vi "Color detection.vi"() -> ()   [LabVIEW 2015]
uses:
  <vilib>/MakerHub/LINX/Public/Peripherals/Digital/Digital Write 1 Chan.vi
  <vilib>/MakerHub/LINX/Public/Peripherals/Digital/Digital Write N Chans.vi
  <vilib>/MakerHub/LINX/Private/Local IO/LinxDigitalWrite.vi
  <vilib>/MakerHub/LINX/Public/Utilities/Check Channel.vi
  <vilib>/MakerHub/LINX/Public/Utilities/Open Serial.vi
  <vilib>/MakerHub/LINX/Private/Utilties/Generate Error.vi
  <vilib>/vision/NI_Vision_Development_Module.lvlib
  <vilib>/MakerHub/LINX/LMH-LINX.lvlib
panel:
  in  "Green OutPin":u8
  in  "Blue Outpin":u8
  in  "Red OutPin":u8
  in  "Serial Port":refnum<visa-resource-name>="N/A"
  out "Green":bool
  out "Blue":bool
  out "Red":bool
  out "Image":T1(plugin-control)
  in  "Rectangle":T2 {"Rotation" min=-90.0 max=90.0 step=1.0 format="%.2f"; "Left" scale=0.0..1024.0; "Right" scale=0.0..1024.0}
  in  "stop":bool
  out "Color Spectrum":dbl[](array[numeric]) format="%.2f"
  in  "Image Type":T3 items=["Grayscale (U8)", "Grayscale (I16)", "Grayscale (SGL)", "Complex (CSG)", "RGB (U32)", "HSL (U32)", "RGB (U64)", "Grayscale (U16)"]
  in  "File Path":path
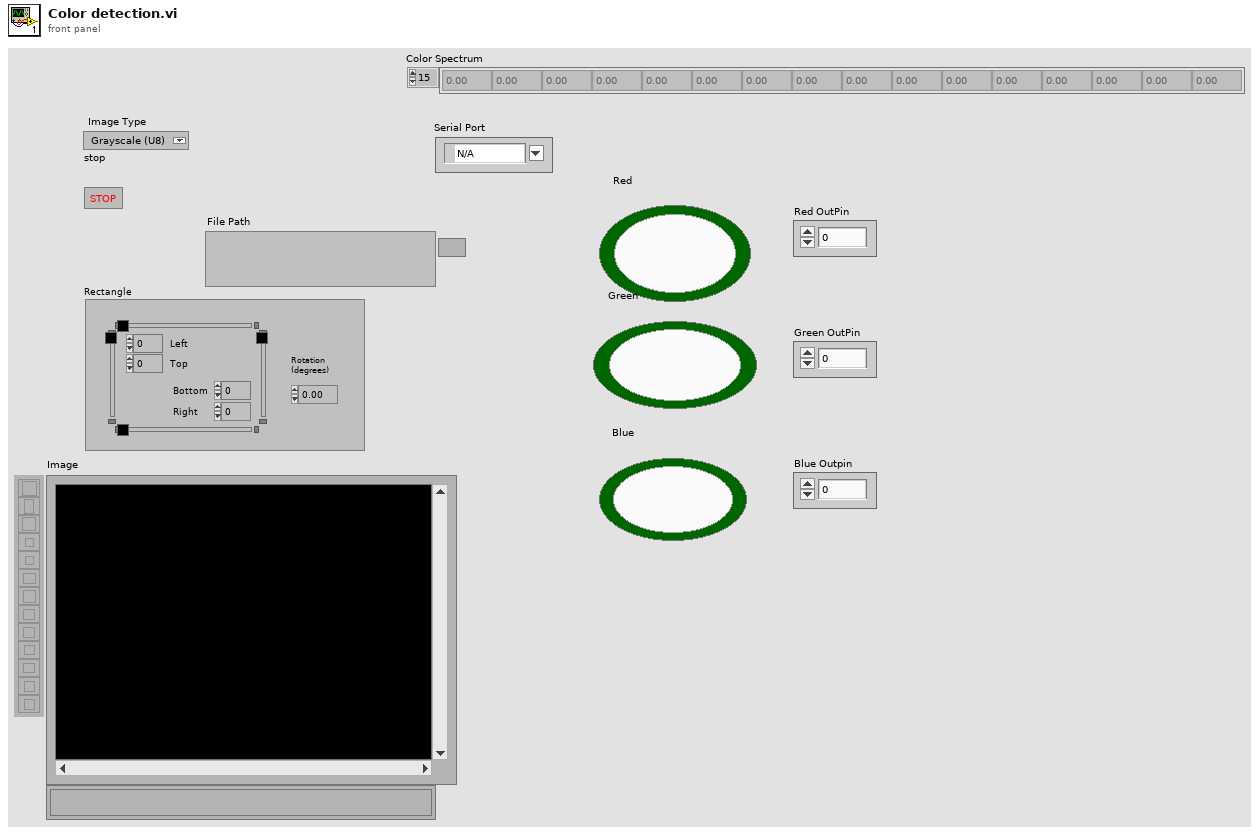
[diagram p1: front panel]
types:
  T1 = typedef "IMAQ Image.ctl" = refnum<image>
  T2 = typedef "IMAQ Rectangle" = cluster{"Left":i32, "Top":i32, "Right":i32, "Bottom":i32, "Rotation":dbl}
  T3 = typedef "Image Type" = u32
  T4 = typedef "LMH-LINX.lvlib/LINX Ref.ctl" = cluster{"IO":T5, "Interface":T6, "LINX Device Config":T7}
  T5 = typedef "LMH-LINX.lvlib/Platform.ctl" = enum16{"Remote", "Local"}
  T6 = typedef "LMH-LINX.lvlib/Interface.ctl" = enum16{"Serial", "TCP"}
  T7 = typedef "LMH-LINX.lvlib/Device.lvlib/LINX Device Config.ctl" = cluster{"Interface":T6, "COM Port":refnum<visa-resource-name>, "TCP Configuration":T8, "Device Family":u8, "Device ID":u8, "Device Name":string, "TCP Ref":refnum<k5>, "Channels":T9}
  T8 = typedef "LMH-LINX.lvlib/Device.lvlib/TCP Config.ctl" = cluster{"IP Address":string, "Port":u16}
  T9 = typedef "LMH-LINX.lvlib/Channels.ctl" = cluster{"DI":u8[], "DO":u8[], "AI":u8[], "AO":u8[], "PWM":u8[], "QE":u8[], "UART":u8[], "I2C 2":u8[], "SPI":u8[], "CAN":u8[], "Servo":u8[], "AI Ref (V)":dbl, "AI Resolution (Bits)":u8, "AO Ref (V)":dbl, "AO Resolution (Bits)":u8}
  T10 = typedef "ROI Descriptor" = cluster{"Global Rectangle":i32[], "Contours":cluster{"ID":enum32{"External", "Internal"}, "Type":u32, "Coordinates":i32[]}[]}
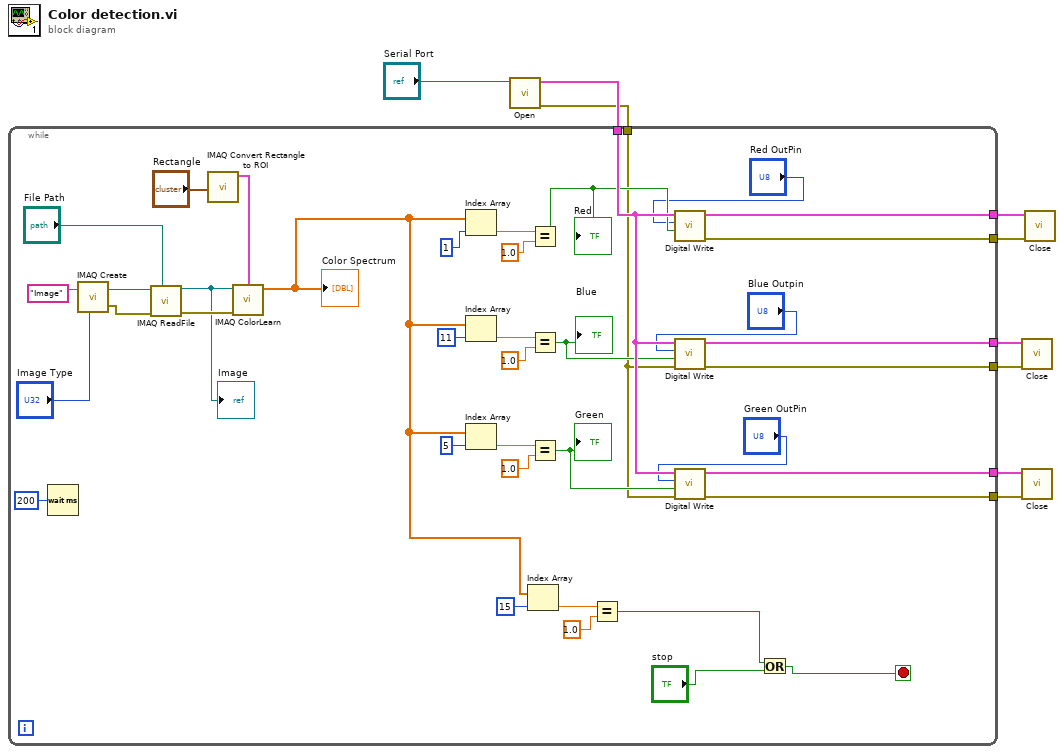
[diagram p0: block diagram]
diagram:
  n1 = call-poly <vilib>:"Open.vi"("Serial Port"="Serial Port") -> ("Error Out"=w7:errorcluster, "LINX Resource"=w8:T4)  [unwired: 8 in, 1 out]
  n2 = while {
    tunnel: w8 -> [w30]
    tunnel: w7 -> [w23]
    tunnel: [w22] -> w6
    tunnel: [w21] -> w5
    tunnel: [w20] -> w4
    tunnel: [w19] -> w3
    tunnel: [w18] -> w2
    tunnel: [w17] -> w1
    stop <- w10 stop-if-true
    n3 = Wait (ms)(milliseconds to wait=u32 200) -> ()  [unwired: 1 out]
    n4 = call "IMAQ Create"("Image Name"="Image", "Image Type"="Image Type") -> ("New Image"=w48:T1, "error out"=w47:errorcluster)  [unwired: 3 in]
    n5 = call "IMAQ ReadFile"("File Path"="File Path", "error in (no error)"=w47, "Image"=w48) -> ("error out"=w43:errorcluster, "Image Out"=w40:T1)  [unwired: 4 in, 3 out]
    "Image" <- w40
    n6 = call "IMAQ Convert Rectangle to ROI"("Rectangle"="Rectangle") -> ("ROI Descriptor"=w42:T10)  [unwired: 8 in, 1 out]
    n7 = call "IMAQ ColorLearn"("ROI Descriptor"=w42, "Image"=w40, "error in (no error)"=w43) -> ("Color Spectrum"=w13:dbl[])  [unwired: 5 in, 1 out]
    "Color Spectrum" <- w13
    n8 = Index Array(array=w13, index=1) -> (element=w38:dbl)
    n9 = Index Array(array=w13, index=11) -> (element=w35:dbl)
    n10 = Index Array(array=w13, index=5) -> (element=w32:dbl)
    n11 = Index Array(array=w13, index=15) -> (element=w15:dbl)
    n12 = Equal?(x=w38, y=1.0) -> (x = y?=w29:bool)
    "Red" <- w29
    n13 = Equal?(x=w35, y=1.0) -> (x = y?=w25:bool)
    "Blue" <- w25
    n14 = Equal?(x=w32, y=1.0) -> (x = y?=w28:bool)
    "Green" <- w28
    n15 = Equal?(x=w15, y=1.0) -> (x = y?=w12:bool)
    n16 = call-poly <vilib>:"Digital Write.vi"("Output Value"=w29, "DO Channel"="Red OutPin", "LINX Resource"=w30) -> ("Error Out"=w21:errorcluster, "LINX Resource"=w22:T4)  [unwired: 7 in]
    n17 = call-poly <vilib>:"Digital Write.vi"("Error In"=w23, "Output Value"=w25, "DO Channel"="Blue Outpin", "LINX Resource"=w30) -> ("Error Out"=w19:errorcluster, "LINX Resource"=w20:T4)  [unwired: 6 in]
    n18 = call-poly <vilib>:"Digital Write.vi"("Error In"=w23, "Output Value"=w28, "DO Channel"="Green OutPin", "LINX Resource"=w30) -> ("Error Out"=w17:errorcluster, "LINX Resource"=w18:T4)  [unwired: 6 in]
    n19 = Or(x=w12, y="stop") -> (x .or. y?=w10:bool)
  }
  n20 = call <vilib>:"Close.vi"("Error In"=w3, "LINX Resource"=w4) -> ()  [unwired: 9 in, 1 out]
  n21 = call <vilib>:"Close.vi"("Error In"=w1, "LINX Resource"=w2) -> ()  [unwired: 9 in, 1 out]
  n22 = call <vilib>:"Close.vi"("Error In"=w5, "LINX Resource"=w6) -> ()  [unwired: 9 in, 1 out]
